vi "Main.vi"() -> ()   [LabVIEW 2012]
doc: "Use this template to build a simple state machine design pattern. Each state executes code and determines which state to transition to."
uses:
  <vilib>/express/express shared/transition.llb/Dynamic To Waveform Array.vi
  <vilib>/express/express shared/transition.llb/Waveform Array To Dynamic.vi
  <vilib>/express/express arith-compare/Formula/Block/exnFormulaBlock how many pts in the wave.vi
  <vilib>/express/express shared/ex_Modify Signal Name.vi
  <vilib>/express/express arith-compare/Formula/XNode/ExpressFormulaBlockNode.xnode
panel:
  in  "Stop Loop?":bool
  out "Pwm Chart":i16(graph)
  out "PWM On":bool
  out "Mass Flow":dbl
  out "Bare, Coated, and DC":T1(graph)
  out "RecCount":i32
  in  "Period (ms)":dbl=3.0
  out "Coated Temperature":dbl
  out "Bare Temperature":dbl
  out "Low Airflow":bool
  in  "Filename to save to":path=path "Z:/adit/Desktop/MEL III/RefrigerationData.lvm" caption="Filename"
  in  "Save Data?":bool=TRUE
  out "Derivative Output":dbl
  out "Integral Output":dbl
  out "CO Bias":dbl
  out "Proportional Output":dbl
  out "Duty Cycle":dbl
  out "Current Set Point":dbl
  in  "Integral Constant":dbl=0.1 caption="I Coefficient" format="%0.2f"
  in  "Derivative \nConstant":dbl=0.05 caption="D Coefficient" format="%0.2f"
  in  "Proportional\nConstant":dbl=1.0 caption="P Coefficient" format="%0.2f"
  in  "Duty Cycle\nincrement amount":dbl=1.0
  in  "Decrease Duty Cycle":bool
  in  "Increase Duty Cycle":bool
  in  "Set Point\nIncrement amount":dbl=1.0
  in  "Lower Set Point":bool
  in  "Raise Set Point":bool
  in  "Bare(T) or \nCoated?":bool
  in  "Manual / Auto":bool
  in  "Time to wait(ms)":u32
  in  "Readings between\nrecorded data":i32
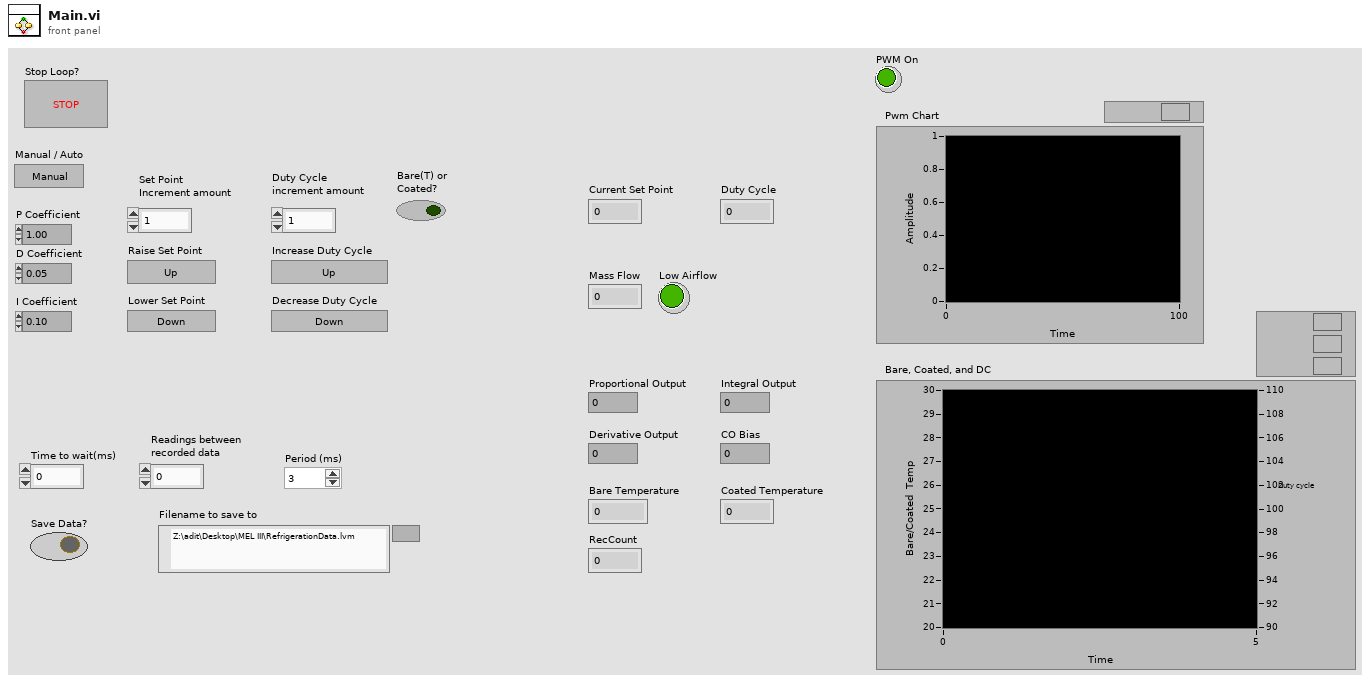
[diagram p1: front panel]
types:
  T1 = cluster{"Uncoated Probe":dbl, "Coated Probe":dbl, "Duty Cycle":dbl}
  T2 = cluster{"RecCount":i32, "Starting Tick Count":i32, "Coated Probe":dbl, "Uncoated Probe":dbl, "Mass Flow":dbl, "Derivative Out":dbl, "Integral Out":dbl, "Proportional Out":dbl, "Manual/Auto":bool, "Set Point":dbl, "Duty Cycle":dbl, "Pwm Value":bool}
  T3 = enum16{"Initialize", "Acquire", "Analyze", "PID", "Record", "PWM", "Output", ""}
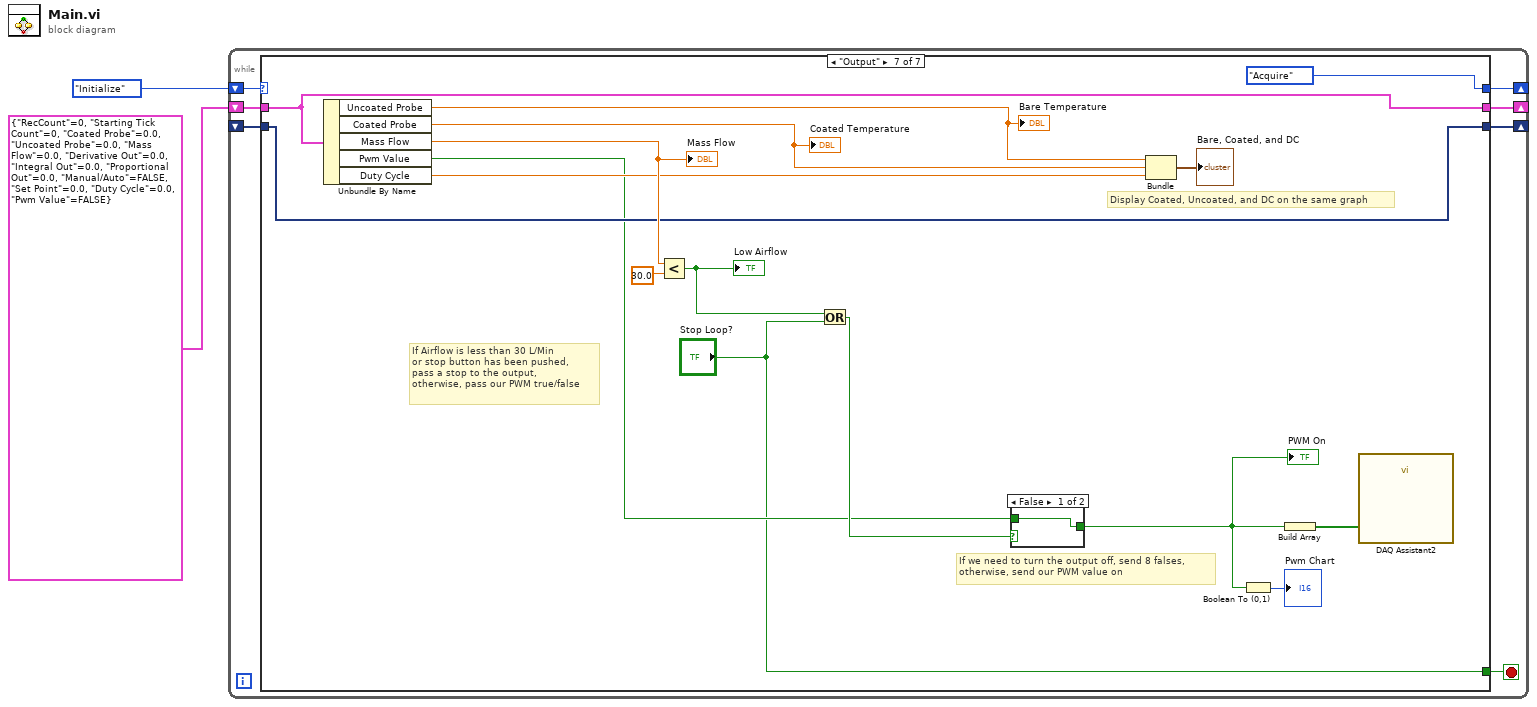
[diagram p0: block diagram]
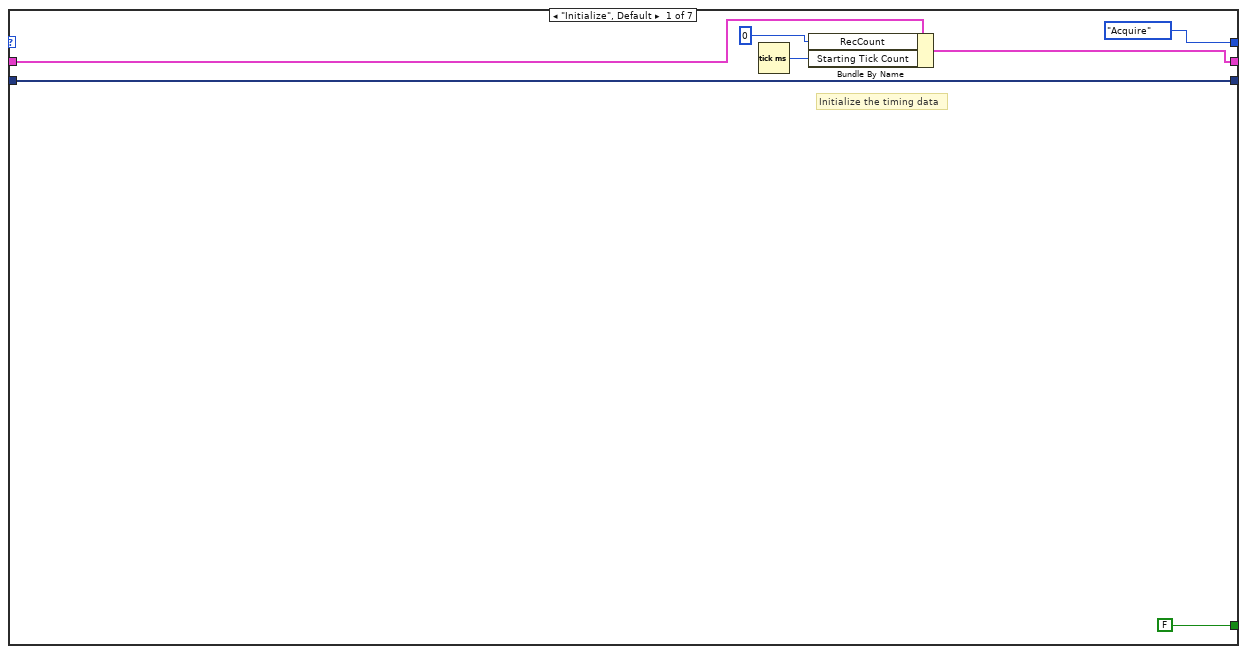
[diagram p2: hidden frame]
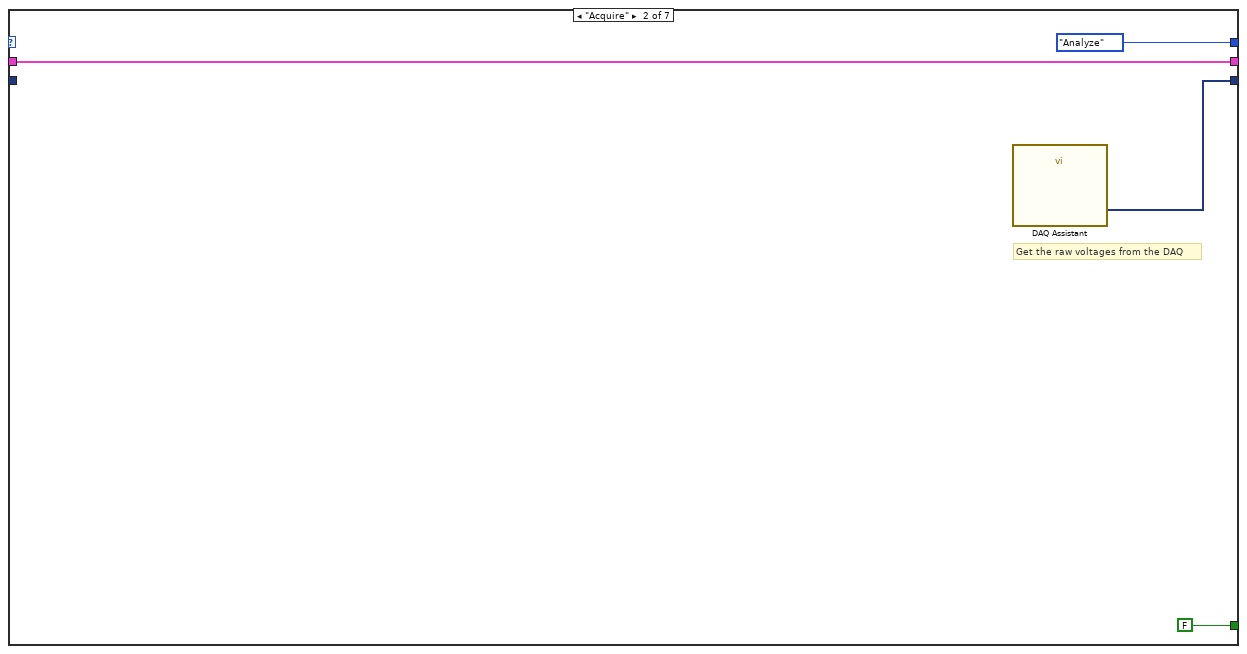
[diagram p3: hidden frame]
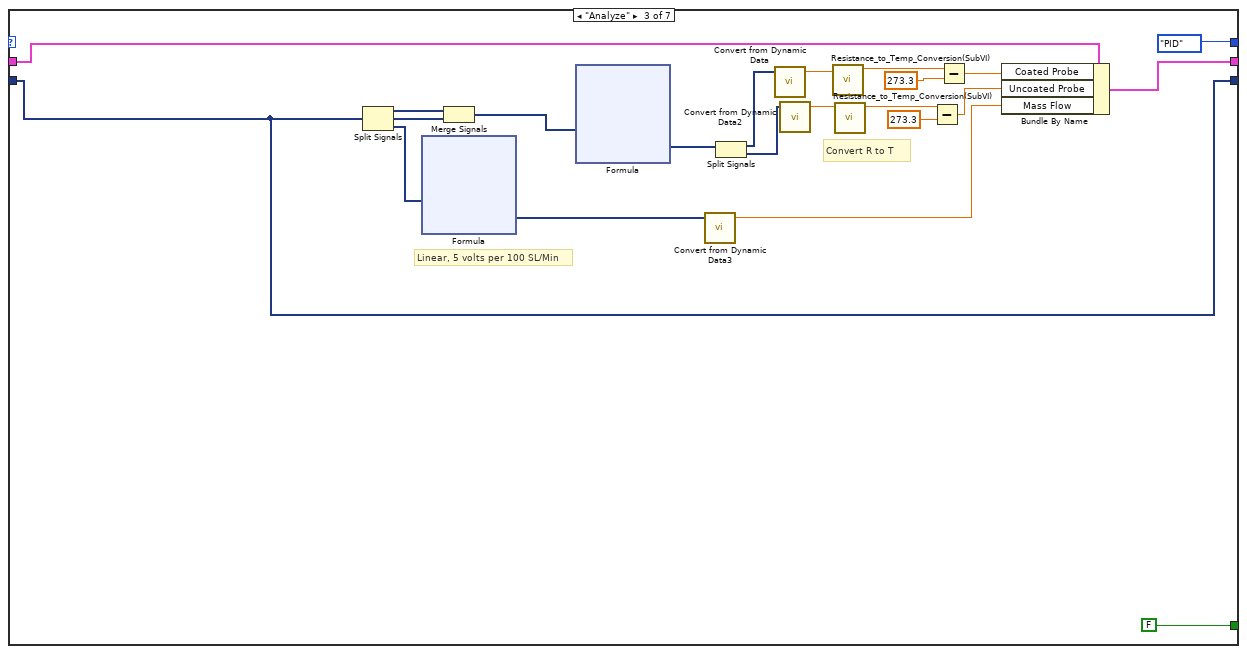
[diagram p4: hidden frame]
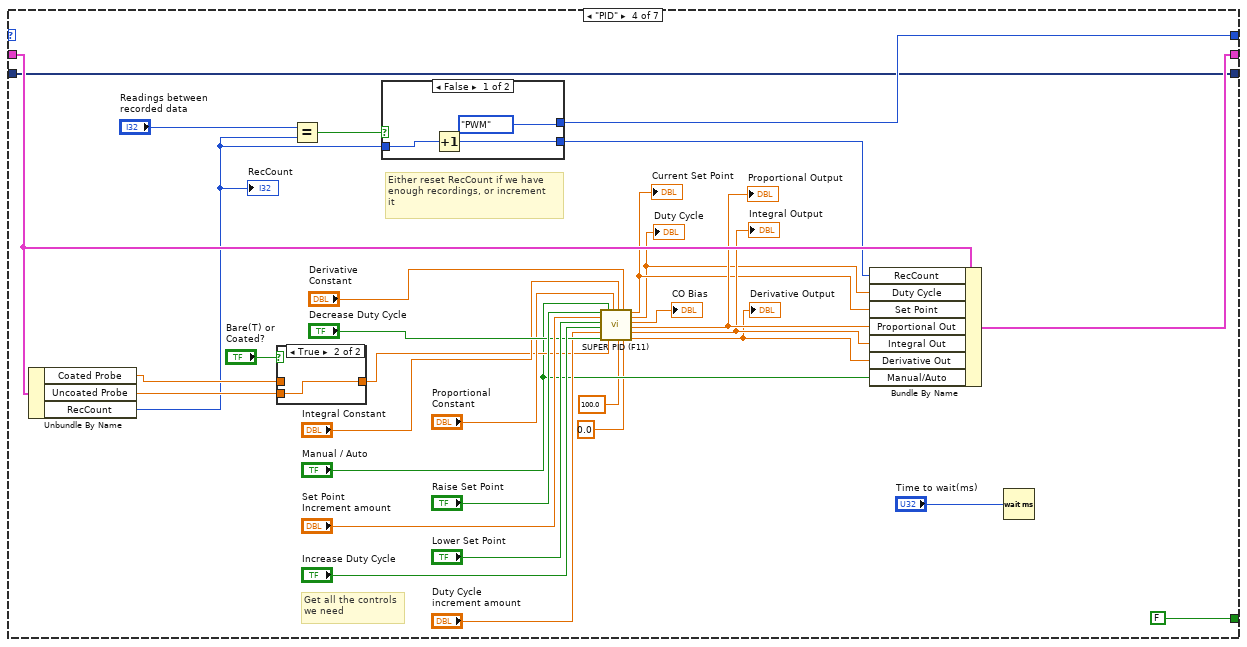
[diagram p5: hidden frame]
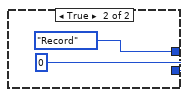
[diagram p7: hidden frame]
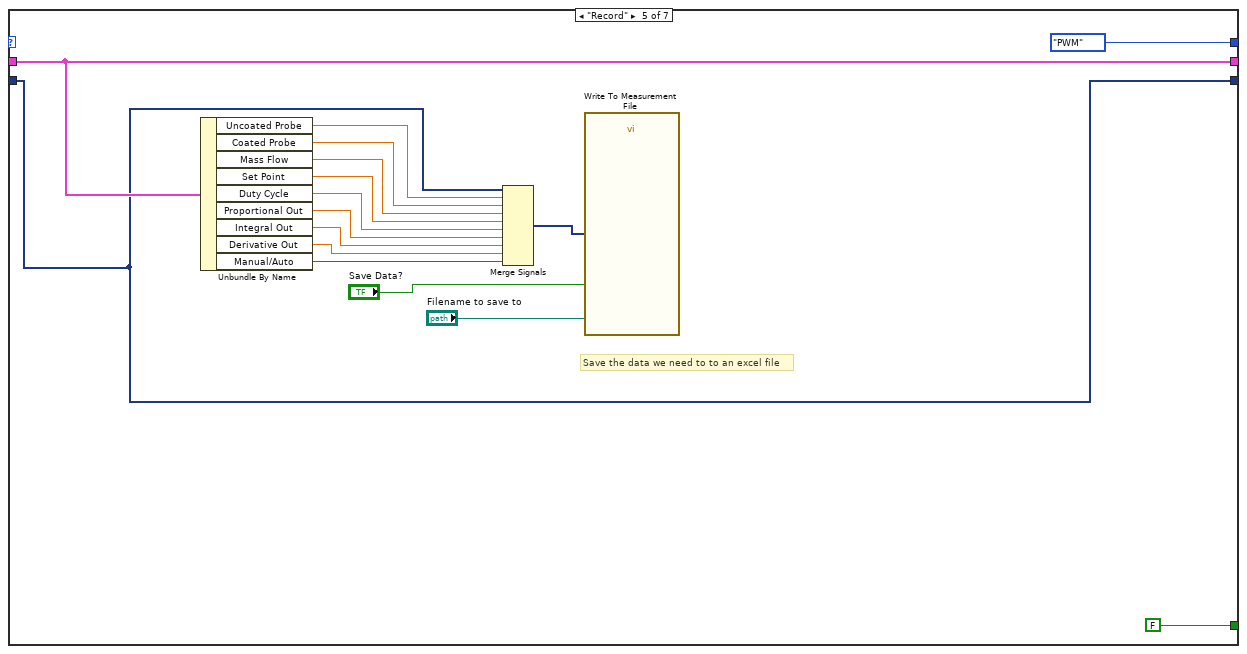
[diagram p8: hidden frame]
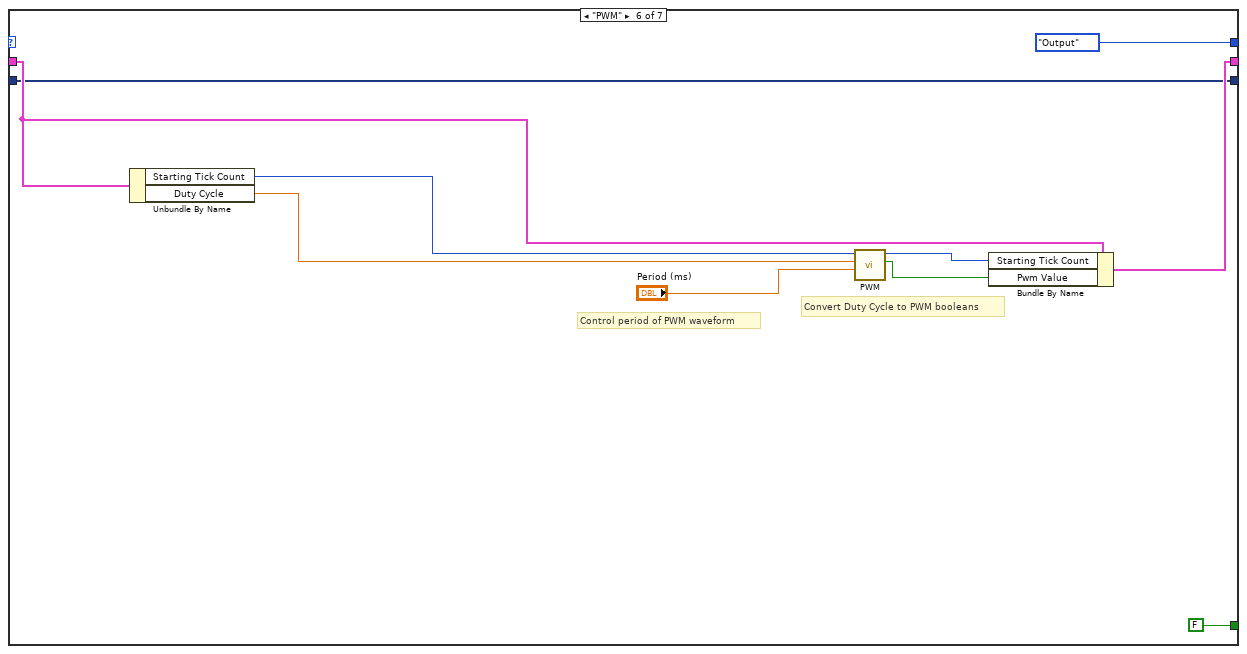
[diagram p9: hidden frame]
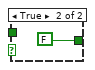
[diagram p10: hidden frame]
diagram:
  n1 = while {
    shift-right: [w8] -> _
    shift-left: T3."Initialize" -> [w9]
    shift-right: [w5] -> _
    shift-left: T2 {"RecCount"=0, "Starting Tick Count"=0, "Coated Probe"=0.0, "Uncoated Probe"=0.0, "Mass Flow"=0.0, "Derivative Out"=0.0, "Integral Out"=0.0, "Proportional Out"=0.0, "Manual/Auto"=FALSE, "Set Point"=0.0, "Duty Cycle"=0.0, "Pwm Value"=FALSE} -> [w6]
    shift-right: [w4] -> _
    shift-left: _ -> [w3]
    stop <- w7 stop-if-true
    n2 = case shown="\"Output\"" w9 {
      tunnel: [T3."Acquire" T3."Analyze" T3."PID" w340 T3."PWM" T3."Output" T3."Acquire"] -> w8
      tunnel: [FALSE FALSE FALSE ("Stop Loop?") FALSE ("Stop Loop?") FALSE FALSE "Stop Loop?"] -> w7
      tunnel: [w13 w18 w32 w330 w361 w380 w398] -> w4
      tunnel: w6 -> [w16 w17 w34 w335 w363 w382 w397]
      tunnel: [w12 w17 w31 w331 w363 w381 w397] -> w5
      tunnel: w3 -> [w13 _ w32 w330 w361 w380 w398]
      frame "Initialize", Default {
        # "Initialize the timing data"
        n3 = Tick Count (ms)() -> (millisecond timer value=w14:u32)
        n4 = Bundle By Name(cluster=w16, "RecCount"=0, "Starting Tick Count"=w14) -> (w12:T2)
      }
      frame "Acquire" {
        # "Get the raw voltages from the DAQ"
        n5 = call "DAQ Assistant"() -> ("data"=w18:dynamicdata)  [unwired: 17 in, 2 out]
      }
      frame "Analyze" {
        # "Linear, 5 volts per 100 SL/Min"
        # "Convert R to T"
        n6 = Split Signals(w32) -> (w37:dynamicdata, w35:dynamicdata, w36:dynamicdata)  [unwired: 3 in]
        n7 = xnode "Formula"("V"=w36) -> ("Result"=w30:dynamicdata)  [unwired: 1 in, 1 out]
        n8 = Merge Signals(w37, w35) -> (w38:dynamicdata)
        n9 = xnode "Formula"("V"=w38) -> ("Result"=w41:dynamicdata)  [unwired: 1 in, 1 out]
        n10 = call "Convert from Dynamic Data3"("Dynamic Data Type"=w30) -> ("Scalar"=w29:dbl)  [unwired: 3 in]
        n11 = Split Signals(w41) -> (w23:dynamicdata, w22:dynamicdata)  [unwired: 2 in]
        n12 = call "Convert from Dynamic Data"("Dynamic Data Type"=w23) -> ("Scalar"=w39:dbl)  [unwired: 3 in]
        n13 = call "Convert from Dynamic Data2"("Dynamic Data Type"=w22) -> ("Scalar"=w40:dbl)  [unwired: 3 in]
        n14 = call "Resistance_to_Temp_Conversion(SubVI).vi"("Scalar"=w39) -> ("Result"=w24:dbl)  [unwired: 10 in]
        n15 = call "Resistance_to_Temp_Conversion(SubVI).vi"("Scalar"=w40) -> ("Result"=w28:dbl)  [unwired: 10 in]
        n16 = Subtract(x=w28, y=273.3) -> (x-y=w27:dbl)
        n17 = Subtract(x=w24, y=273.3) -> (x-y=w21:dbl)
        n18 = Bundle By Name(cluster=w34, "Coated Probe"=w21, "Uncoated Probe"=w27, "Mass Flow"=w29) -> (w31:T2)
      }
      frame "PID" {
        # "Either reset RecCount if we have\nenough recordings, or increment\nit"
        # "Get all the controls\nwe need"
        n19 = Unbundle By Name(w335) -> ("Coated Probe"=w333:dbl, "Uncoated Probe"=w336:dbl, "RecCount"=w332:i32)
        "RecCount" <- w332
        n20 = case shown="True" "Bare(T) or \nCoated?" {
          tunnel: w333 -> [w353 _]
          tunnel: w336 -> [_ w354]
          tunnel: [w353 w354] -> w337
          frame False {
          }
          frame True {
          }
        }
        n21 = Equal?(x="Readings between\nrecorded data", y=w332) -> (x = y?=w342:bool)
        n22 = case shown="False" w342 {
          tunnel: [T3."PWM" T3."Record"] -> w340
          tunnel: [w356 0] -> w334
          tunnel: w332 -> [w355 _]
          frame False {
            n23 = Increment(x=w355) -> (x+1=w356:i32)
          }
          frame True {
          }
        }
        n24 = call "SUPER PID (F11).vi"("SP Up"="Raise Set Point", "SP Increment"="Set Point\nIncrement amount", "SP Down"="Lower Set Point", "DC Up"="Increase Duty Cycle", "DC Increment"="Duty Cycle\nincrement amount", "DC Down"="Decrease Duty Cycle", "Manual / Auto"="Manual / Auto", "PV"=w337, "P"="Proportional\nConstant", "I"="Integral Constant", "upper limit"=100.0, "D"="Derivative \nConstant", "lower limit"=0.0) -> ("SP"=w325:dbl, "DC"=w324:dbl, "CO Bias"=→"CO Bias":dbl, "P out"=w329:dbl, "I out"=w328:dbl, "D out"=w327:dbl)  [unwired: 1 in]
        "Current Set Point" <- w325
        "Duty Cycle" <- w324
        "Proportional Output" <- w329
        "Integral Output" <- w328
        "Derivative Output" <- w327
        n25 = Bundle By Name(cluster=w335, "RecCount"=w334, "Duty Cycle"=w324, "Set Point"=w325, "Proportional Out"=w329, "Integral Out"=w328, "Derivative Out"=w327, "Manual/Auto"="Manual / Auto") -> (w331:T2)
        n26 = Wait (ms)(milliseconds to wait="Time to wait(ms)") -> ()  [unwired: 1 out]
      }
      frame "Record" {
        # "Save the data we need to to an excel file"
        n27 = Unbundle By Name(w363) -> ("Uncoated Probe"=w362:dbl, "Coated Probe"=w373:dbl, "Mass Flow"=w372:dbl, "Set Point"=w365:dbl, "Duty Cycle"=w371:dbl, "Proportional Out"=w370:dbl, "Integral Out"=w364:dbl, "Derivative Out"=w367:dbl, "Manual/Auto"=w366:bool)
        n28 = Merge Signals(w361, w362, w373, w372, w365, w371, w370, w364, w367, w366) -> (w374:dynamicdata)
        n29 = call "Write To Measurement File"("Signals"=w374, "Enable"="Save Data?", "Filename"="Filename to save to") -> ()  [unwired: 14 in, 3 out]
      }
      frame "PWM" {
        # "Control period of PWM waveform"
        # "Convert Duty Cycle to PWM booleans"
        n30 = Unbundle By Name(w382) -> ("Starting Tick Count"=w378:i32, "Duty Cycle"=w383:dbl)
        n31 = call "PWM.vi"("Period (ms)"="Period (ms)", "Duty Cycle"=w383, "Starting Tick Count"=w378) -> ("Pwm value"=w376:bool, "Starting Tick Count"=w377:u32)  [unwired: 7 in]
        n32 = Bundle By Name(cluster=w382, "Starting Tick Count"=w377, "Pwm Value"=w376) -> (w381:T2)
      }
      frame "Output" {
        # "If we need to turn the output off, send 8 falses, \notherwise, send our PWM value on"
        # "Display Coated, Uncoated, and DC on the same graph"
        # "If Airflow is less than 30 L/Min\nor stop button has been pushed, \npass a stop to the output,\notherwise, pass our PWM true/false"
        n33 = Unbundle By Name(w397) -> ("Uncoated Probe"=w395:dbl, "Coated Probe"=w394:dbl, "Mass Flow"=w400:dbl, "Pwm Value"=w391:bool, "Duty Cycle"=w393:dbl)
        "Bare Temperature" <- w395
        "Coated Temperature" <- w394
        "Mass Flow" <- w400
        n34 = Less?(x=w400, y=30.0) -> (x < y?=w387:bool)
        "Low Airflow" <- w387
        n35 = Or(x=w387, y="Stop Loop?") -> (x .or. y?=w399:bool)
        n36 = case shown="False" w399 {
          tunnel: [w402 FALSE] -> w388
          tunnel: w391 -> [w402 _]
          frame False {
          }
          frame True {
          }
        }
        "PWM On" <- w388
        n37 = Bundle("Uncoated Probe"=w395, "Coated Probe"=w394, "Duty Cycle"=w393) -> (→"Bare, Coated, and DC":T1)  [unwired: 1 in]
        n38 = Boolean To (0,1)(Boolean=w388) -> (0, 1=→"Pwm Chart":i16)
        n39 = Build Array(w388) -> (w389:bool[])
        n40 = call "DAQ Assistant2"("data"=w389) -> ()  [unwired: 17 in, 2 out]
      }
    }
  }
